vi "Read Results from processing.vi"(8 "error in":errorcluster, 11 "State Machine runtime in":refnum<class "State Machine runtime.lvclass">) -> (0 "error out":errorcluster, 2 "Results from processing":T1, 3 "State Machine runtime out":refnum<class "State Machine runtime.lvclass">)   [LabVIEW 2021, in "State Machine runtime.lvclass"]
uses:
  State Machine runtime.lvclass
  configuration/result data indices.ctl
  State Machine runtime.lvclass/State Machine runtime.ctl
  configuration/State Machine configuration.lvclass
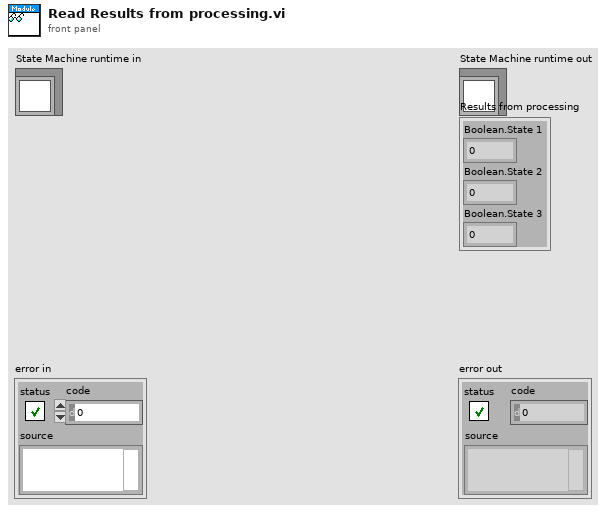
[diagram p1: front panel]
types:
  T1 = typedef "State Machine configuration.lvclass/result data indices.ctl" = cluster{"Boolean.State 1":i32, "Boolean.State 2":i32, "Boolean.State 3":i32}
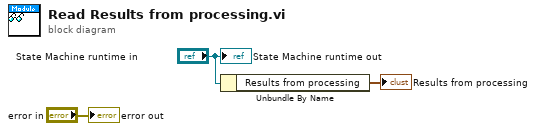
[diagram p0: block diagram]
diagram:
  n1 = Unbundle By Name("State Machine runtime in") -> ("Results from processing"=→"Results from processing":T1)
  "error out" <- "error in"
  "State Machine runtime out" <- "State Machine runtime in"
